vi "Acquisition & Generation (Amplitude Reg) test.vi"() -> ()   [LabVIEW 2014]
uses:
  <vilib>/Platform/TimedLoop/XDataNode/timing_clust.ctl
  <vilib>/Platform/TimedLoop/XDataNode/nitl_modes.ctl
  <vilib>/Platform/TimedLoop/XDataNode/wakeup.ctl
  <vilib>/rvi/Emulation/niFpgaSctlEmulationGetInTimedLoop.vi
  <vilib>/rvi/Emulation/niFpgaEmulationReportErrorSimple.vi
  <vilib>/rvi/Emulation/niFpgaGetClockAttributes.vi
  <vilib>/rvi/Emulation/niFpgaCriticalErrorInLSC.vi
  <vilib>/rvi/Memory/Memory_Emulation/nirvimemoryFastEmulation.vi
  <vilib>/rvi/Memory/Memory_Emulation/nirvimemoryEmulation.vi
  <vilib>/rvi/Emulation/niFpgaEmulationIsFPGAContextNoSignature.vi
  <vilib>/rvi/DataTransferAndStorage/Container/Common/niFpgaContainerGetUniqueNameForEmu.vi
  <vilib>/rvi/Emulation/niFpgaProcessEmulError.vi
  <vilib>/rvi/errors/nirviReportUnexpectedCaseInternalError (U32).vi
  <vilib>/rvi/errors/niFpgaSetErrorForExecOnDevCompSimple.vi
  <vilib>/rvi/eio/common/nirviEmuReportErrorAndStop.vi
  <vilib>/rvi/FIFO/Fifo_Resource/nirvififoEmulationSetSize.vi
  <vilib>/rvi/FIFO/Fifo_Resource/nirviFifoEmulationQueueMgr.vi
  <instcachedir>/0/nirviFifoEmulationQueueMgr_E5CAEC123FF24DC58D834DCA3CDAA9B5.lvgen/nirviFifoEmulationQueueMgr_E5CAEC123FF24DC58D834DCA3CDAA9B5_010.vi
  <vilib>/rvi/FIFO/Fifo_Resource/nirvififoEmulationDetermineInputValidOut.vi
  <vilib>/rvi/FIFO/Fifo_Resource/nirvififoEmulationCreateLock.vi
  <vilib>/rvi/FIFO/Fifo_Resource/nirvififoEmulationObtainLock.vi
  <vilib>/rvi/FIFO/Fifo_Resource/nirvififoEmulationReleaseLock.vi
  <vilib>/rvi/occurrence/nirviWaitOnOccurrenceBase.vi
  <vilib>/rvi/errors/nirviReportUnexpectedCaseInternalError.vi
  <vilib>/rvi/interface/RandomDataEmulation/niFpgaRandomDataHandleErrors.vi
  <vilib>/rvi/eio/common/nirviEmuTemplateMethod_errors.vi
  <vilib>/Platform/TimedLoop/XDataNode/XDataNode.xnode
  <vilib>/rvi/DataTransferAndStorage/Container/XNode/niFpgaContainer.xnode
  <vilib>/rvi/FIFO/Fifo_Resource/nirvififoEmulationWrite.vi
  <vilib>/rvi/interface/RandomDataEmulation/nirviRandomDataFpgaReadWriteTemplate.vi
  <vilib>/rvi/FIFO/Fifo_Resource/nirvififoEmulationRead.vi
  <vilib>/eio/EIOMethodNode/EIOMethodNode.xnode
  <vilib>/Platform/TimedLoop/XDataNode/XDNodeRunTimeDep.lvlib
panel:
  out "Waveform Chart":i16(graph)
  in  "Amplitude (0:1)":fxp<+,4,1>=1.0
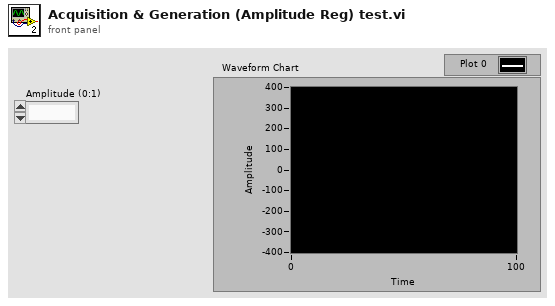
[diagram p1: front panel]
types:
  T1 = typedef "XDNodeRunTimeDep.lvlib/timing_clust.ctl" = cluster{"Expected End [f-1]":u64, "Actual End [f-1]":u64, "Finished Late? [f-1]":bool, "Expected End [i-1]":u64, "Actual End [i-1]":u64, "Finished Late? [i-1]":bool, "Expected Start [i]":u64, "Actual Start [i]":u64, "Expected Start [f]":u64, "Actual Start [f]":u64, "Source Name":string, "Structure Name":string, "Period":i64, "Deadline":i64, "Offset":i64, "Start":i64, "Priority":i32, "Timeout":i32, "Mode":T2, "Wakeup Reason":T3, "Error":errorcluster, "Source Type":string, "Secondary Source Type":string, "Global End Time":u64, "Global Start Time":u64, "Frame Duration":u64, "Iteration Duration":u64, "Assigned CPU":i32, "I/O Scan Engine Mode":u32}
  T2 = typedef "XDNodeRunTimeDep.lvlib/nitl_modes.ctl" = enum32{"No Change", "Process missed periods, maintain original phase", "Discard missed periods, maintain original phase", "Process missed periods, ignore original phase", "Discard missed periods, ignore original phase"}
  T3 = typedef "XDNodeRunTimeDep.lvlib/wakeup.ctl" = enum32{"Normal", "Aborted", "Asynchronous wakeup", "Timing source error", "Timed loop error", "Timeout"}
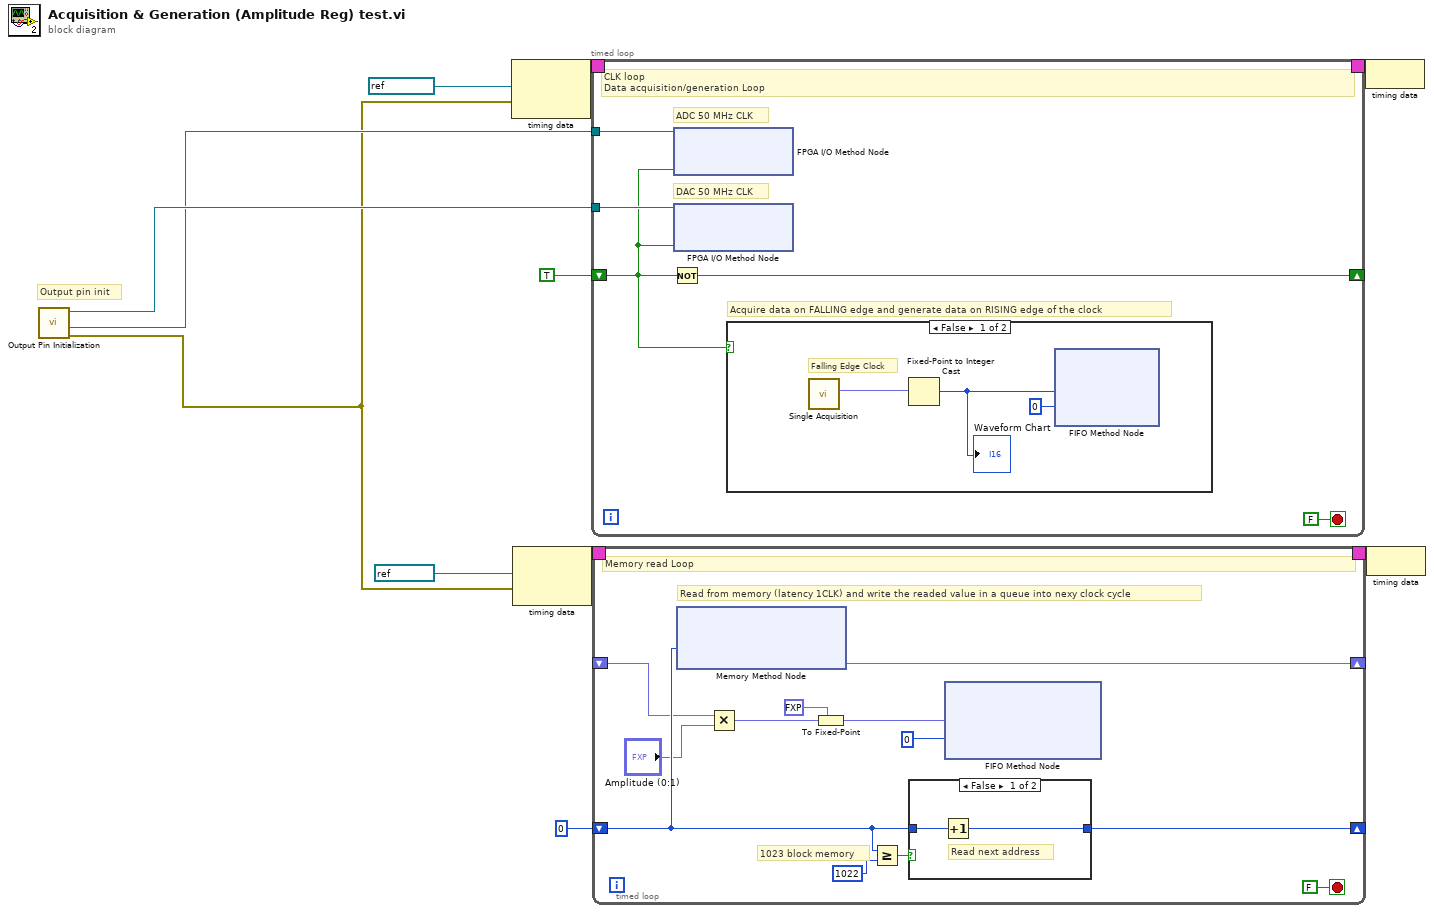
[diagram p0: block diagram]
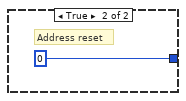
[diagram p2: hidden frame]
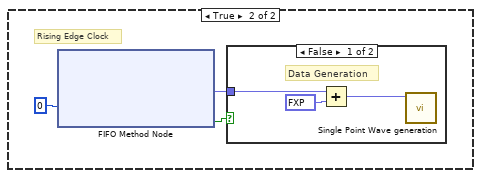
[diagram p3: hidden frame]
diagram:
  # "Output pin init"
  n1 = call "Output Pin Initialization.vi"() -> ("error out"=w1:errorcluster, "I/O Out Clock DAC (pin16)"=w2:refnum<k21>, "I/O Out Clock ADC (pin17)"=w3:refnum<k21>)  [unwired: 8 in]
  n2 = node-c288(refnum<k21> "100MHz" ("Source Name"), w1) -> (w11:T1)
  n3 = node-c288(refnum<k21> "50MHz" ("Source Name"), w1) -> (w9:T1)
  n4 = timed-loop {
    timing: w11 -> [_]
    timing-out: [_] -> w10
    shift-right: [w14] -> _
    shift-left: TRUE -> [w12]
    tunnel: w2 -> [w16]
    tunnel: w3 -> [w13]
    stop <- FALSE stop-if-true
    # "DAC 50 MHz CLK"
    # "Acquire data on FALLING edge and generate data on RISING edge of the clock"
    # "ADC 50 MHz CLK"
    # "CLK loop\nData acquisition/generation Loop"
    n5 = Not(x=w12) -> (.not. x?=w14:bool)
    n6 = xnode "FPGA I/O Method Node"("FPGA I/O In"=w16, "Data"=w12) -> ()  [unwired: 1 out]
    n7 = xnode "FPGA I/O Method Node"("FPGA I/O In"=w13, "Data"=w12) -> ()  [unwired: 1 out]
    n8 = case shown="False" w12 {
      frame False {
        # "Falling Edge Clock"
        n9 = call "Single Acquisition.vi"() -> ("Out"=w17:fxp<+/-,12,12>)  [unwired: 10 in, 1 out]
        n10 = Fixed-Point to Integer Cast(1:w17) -> (0:w18:i16)
        "Waveform Chart" <- w18
        n11 = xnode ("FIFO Method Node")("Element"=w18, "Timeout"=0) -> ()  [unwired: 1 in, 2 out]
      }
      frame True {
        # "Rising Edge Clock"
        n12 = xnode ("FIFO Method Node")("Timeout"=0) -> ("Element"=w20:fxp<+/-,12,12>, "Timed Out?"=w21:bool)  [unwired: 1 in, 1 out]
        n13 = case shown="False" w21 {
          tunnel: w20 -> [w25 _]
          frame False {
            # "Data Generation"
            n14 = Add(x=w25, y=fxp<+,12,12> 2048.0) -> (x+y=w23:fxp<+/-,14,14>)
            n15 = call "Single Point Wave generation.vi"("Data To Write"=w23) -> ()  [unwired: 10 in, 1 out]
          }
          frame True {
            # "FPGA memory slow"
          }
        }
      }
    }
  }
  n16 = timed-loop {
    timing: w9 -> [_]
    timing-out: [_] -> w8
    shift-right: [w39] -> _
    shift-left: _ -> [w29]
    shift-right: [w36] -> _
    shift-left: u32 0 -> [w33]
    stop <- FALSE stop-if-true
    # "1023 block memory"
    # "Read from memory (latency 1CLK) and write the readed value in a queue into nexy clock cycle"
    # "Memory read Loop"
    n17 = xnode ("Memory Method Node")("Address"=w33) -> ("Data"=w39:fxp<+/-,12,12>)  [unwired: 1 in, 1 out]
    n18 = Multiply(x=w29, y="Amplitude (0:1)") -> (x*y=w31:fxp<+/-,16,13>)
    n19 = To Fixed-Point(fixed-point type=fxp<+/-,12,12> 0.0, number=w31) -> (fixed-point=w30:fxp<+/-,12,12>)
    n20 = Greater Or Equal?(x=w33, y=u32 1022) -> (x >= y?=w37:bool)
    n21 = case shown="False" w37 {
      tunnel: w33 -> [w41 _]
      tunnel: [w40 u32 0] -> w36
      frame False {
        # "Read next address"
        n22 = Increment(x=w41) -> (x+1=w40:u32)
      }
      frame True {
        # "Address reset"
      }
    }
    n23 = xnode ("FIFO Method Node")("Element"=w30, "Timeout"=0) -> ()  [unwired: 1 in, 2 out]
  }
  n24 = node-c288(w10) -> ()
  n25 = node-c288(w8) -> ()
